vi "Triangle Search.vi"(0 "X":dbl[](array[numeric]), 5 "Y":dbl[](array[numeric]), 7 "Triangles":i32[][](array[numeric]), 9 "Xi":dbl[](array[numeric]), 11 "Yi":dbl[](array[numeric])) -> (8 "indices":dbl[](array[numeric]), 15 "error":i32)   [LabVIEW 2017, in "NI_AAL_Geometry.lvlib"]
uses:
  <vilib>/Analysis/NI_AAL_Geometry.lvlib
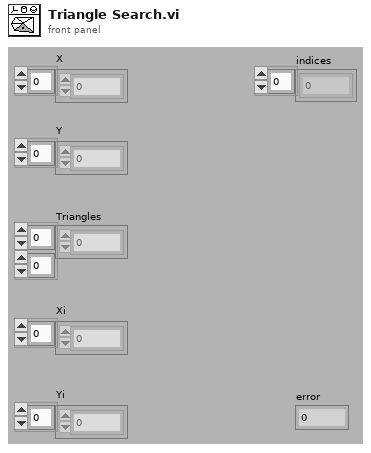
[diagram p1: front panel]
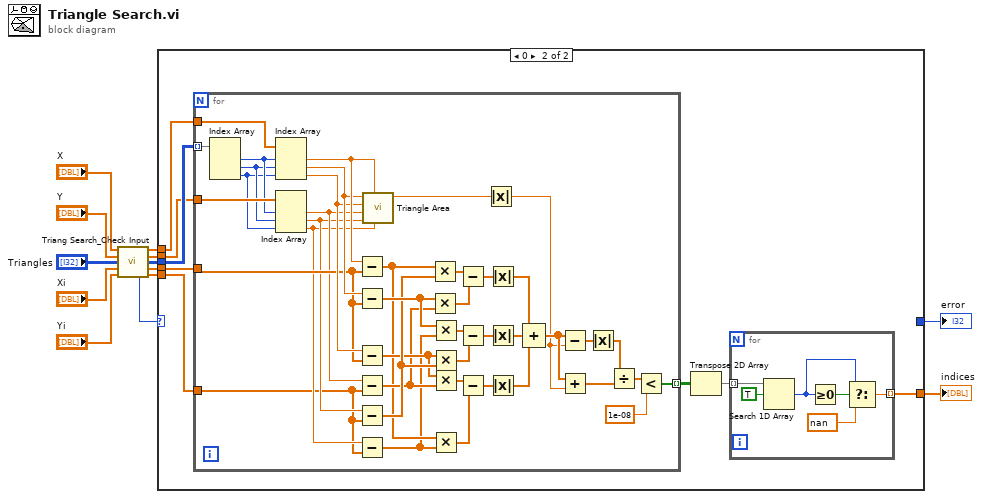
[diagram p0: block diagram]
diagram:
  n1 = call <vilib>:"Triang Search_Check Input.vi"("X In"="X", "Y In"="Y", "Triangles In"="Triangles", "Xi"="Xi", "Yi"="Yi") -> ("X Out"=w10:dbl[], "Y Out"=w8:dbl[], "Triangles Out"=w2:i32[][], "Xi Out"=w6:dbl[], "error"=w12:i32, "Yi Out"=w4:dbl[])  [unwired: 5 out]
  n2 = case shown="0" w12 {
    selector: w12 -> [w14 _]
    tunnel: [_ w15] -> w13
    tunnel: w10 -> [_ w16]
    tunnel: w8 -> [_ w17]
    tunnel: w2 -> [_ w20]
    tunnel: w6 -> [_ w19]
    tunnel: w4 -> [_ w18]
    tunnel: [w14 _] -> w1
    frame -1, Default {
    }
    frame 0 {
      n3 = for {
        tunnel: w20 -> [w69] mode=indexing
        tunnel: w17 -> [w67]
        tunnel: w16 -> [w68]
        tunnel: w19 -> [w60]
        tunnel: w18 -> [w56]
        tunnel: [w29] -> w22 mode=indexing
        n4 = Index Array(array=w69) -> (element #1=w66:i32, element #2=w65:i32, element #3=w64:i32)  [unwired: 3 in]
        n5 = Index Array(array=w68, index #1=w66, index #2=w65, index #3=w64) -> (element #1=w63:dbl, element #2=w62:dbl, element #3=w61:dbl)
        n6 = Index Array(array=w67, index #1=w66, index #2=w65, index #3=w64) -> (element #1=w59:dbl, element #2=w58:dbl, element #3=w57:dbl)
        n7 = Subtract(x=w63, y=w60) -> (x-y=w45:dbl[])
        n8 = Subtract(x=w62, y=w60) -> (x-y=w53:dbl[])
        n9 = Subtract(x=w61, y=w60) -> (x-y=w47:dbl[])
        n10 = Subtract(x=w59, y=w56) -> (x-y=w46:dbl[])
        n11 = Subtract(x=w58, y=w56) -> (x-y=w52:dbl[])
        n12 = Subtract(x=w57, y=w56) -> (x-y=w44:dbl[])
        n13 = call <vilib>:"Triangle Area.vi"("y 3"=w57, "x 1"=w63, "y 2"=w58, "y 1"=w59, "x 3"=w61, "x 2"=w62) -> ("area"=w40:dbl)  [unwired: 5 in]
        n14 = Multiply(x=w45, y=w52) -> (x*y=w55:dbl[])
        n15 = Multiply(x=w53, y=w46) -> (x*y=w54:dbl[])
        n16 = Multiply(x=w53, y=w44) -> (x*y=w51:dbl[])
        n17 = Multiply(x=w47, y=w52) -> (x*y=w50:dbl[])
        n18 = Multiply(x=w47, y=w46) -> (x*y=w48:dbl[])
        n19 = Multiply(x=w45, y=w44) -> (x*y=w49:dbl[])
        n20 = Subtract(x=w55, y=w54) -> (x-y=w43:dbl[])
        n21 = Subtract(x=w51, y=w50) -> (x-y=w42:dbl[])
        n22 = Subtract(x=w48, y=w49) -> (x-y=w41:dbl[])
        n23 = Absolute Value(x=w40) -> (abs(x)=w30:dbl)
        n24 = Absolute Value(x=w43) -> (abs(x)=w39:dbl[])
        n25 = Absolute Value(x=w42) -> (abs(x)=w38:dbl[])
        n26 = Absolute Value(x=w41) -> (abs(x)=w37:dbl[])
        n27 = Compound Arithmetic op=ADD(w39, w38, w37) -> (w31:dbl[])
        n28 = Subtract(x=w31, y=w30) -> (x-y=w36:dbl[])
        n29 = Add(x=w31, y=w30) -> (x+y=w34:dbl[])
        n30 = Absolute Value(x=w36) -> (abs(x)=w33:dbl[])
        n31 = Divide(x=w33, y=w34) -> (x/y=w32:dbl[])
        n32 = Less?(x=w32, y=1e-08) -> (x < y?=w29:bool[])
      }
      n33 = Transpose 2D Array(2D array=w22) -> (transposed array=w21:bool[][])
      n34 = for {
        tunnel: w21 -> [w28] mode=indexing
        tunnel: [w23] -> w15 mode=indexing
        n35 = Search 1D Array(1D array=w28, element=TRUE) -> (index of element=w25:i32)  [unwired: 1 out]
        n36 = Greater Or Equal To 0?(x=w25) -> (x >= 0?=w24:bool)
        n37 = Select(t=w25, s=w24, f=nan) -> (s? t:f=w23:dbl)
      }
    }
  }
  "indices" <- w13
  "error" <- w1
